vi "Song Generator.vi"() -> ()   [LabVIEW 2014]
panel:
  in  "Song":T1(array[cluster])=[{"frequency (Hz)"=328, "duration (msec)"=1000}, {"frequency (Hz)"=292, "duration (msec)"=1000}, {"frequency (Hz)"=261, "duration (msec)"=1000}, {"frequency (Hz)"=294, "duration (msec)"=1000}, {"frequency (Hz)"=332, "duration (msec)"=507}, {"frequency (Hz)"=332, "duration (msec)"=489}, {"frequency (Hz)"=328, "duration (msec)"=508}] {"duration (msec)" scale=200.0..1000.0; "frequency (Hz)" scale=261.0..523.0}
  # "C\nB\nA\nG\nF\nE\nD\nC"
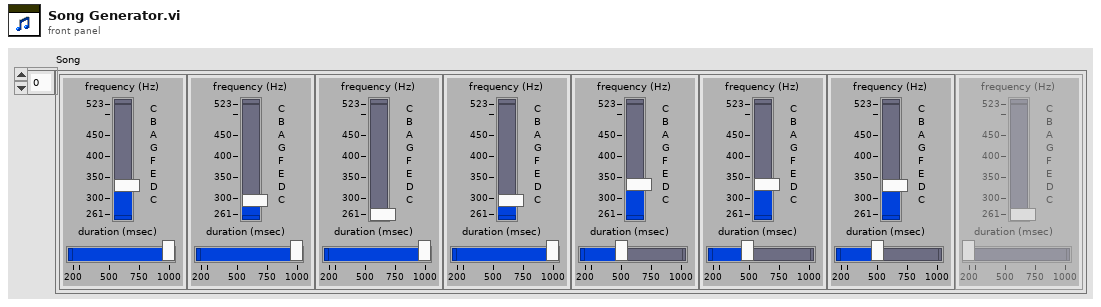
[diagram p1: front panel]
types:
  T1 = cluster{"frequency (Hz)":u32, "duration (msec)":u32}[]
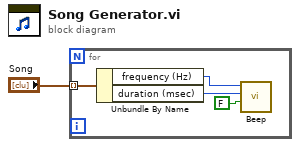
[diagram p0: block diagram]
diagram:
  n1 = for {
    tunnel: "Song" -> [w4] mode=indexing
    n2 = Unbundle By Name(w4) -> ("frequency (Hz)"=w3:u32, "duration (msec)"=w2:u32)
    n3 = call <vilib>:"Beep.vi"("use system alert? (T)"=FALSE, "duration (msec)"=w2, "frequency (Hz)"=w3) -> ()  [unwired: 9 in]
  }
